vi "UE9 Frequency Output Stepping.vi"(8 "error in":errorcluster) -> (0 "error out":errorcluster)   [LabVIEW 2021]
panel:
  in  "Run Continuously":bool
  in  "Step Up and Down":bool
  out "Current Frequency":dbl=1.0 format="%.2f"
  in  "ms at each step":dbl=1000.0 format="%.2f"
  in  "stop":bool
  in  "Step Size":dbl=2000.0 format="%.2f"
  in  "Finish Frequency":dbl=10000.0 format="%.2f"
  in  "Start Frequency":dbl=2000.0 format="%.2f"
  in  "FirstFound":bool=TRUE
  in  "Address":string="1"
  in  "ConnectionType":u16(ring) items=["LJ_ctUSB", "LJ_ctETHERNET"]
  out "Error Message":string
  # "Demonstrates 1 channel of frequency output sweeping on FIO0."
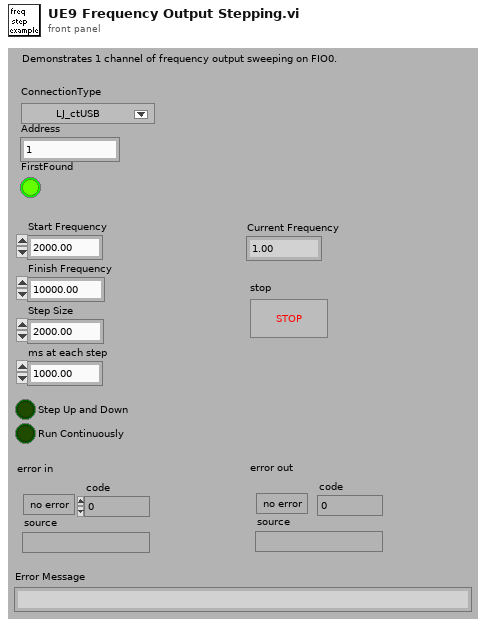
[diagram p1: front panel]
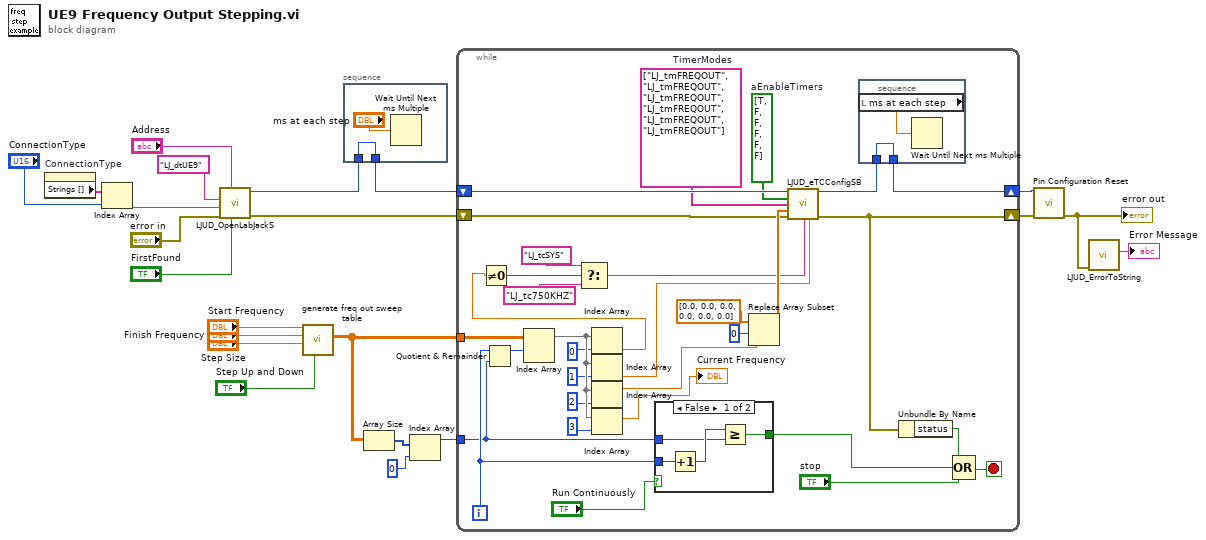
[diagram p0: block diagram]
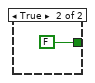
[diagram p2: hidden frame]
diagram:
  n1 = property on="ConnectionType" class="Ring (strict)"() -> ("Strings []"=w8:string[])  [unwired: 2 in, 2 out]
  n2 = Index Array(array=w8, index="ConnectionType") -> (element=w7:string)
  n3 = call "LJUD_OpenLabJackS.vi"("FirstFound"="FirstFound", "Address"="Address", "error in"="error in", "ConnectionType"=w7, "DeviceType"="LJ_dtUE9") -> ("error out"=w1:errorcluster, "Handle"=w2:i32)  [unwired: 4 in, 1 out]
  n4 = call "generate freq out sweep table.vi"("Step Up and Down"="Step Up and Down", "Step Size"="Step Size", "Finish Frequency"="Finish Frequency", "Start Frequency"="Start Frequency") -> ("Clock, ClockDivisor, FreqDivisor, Frequency"=w15:dbl[][])  [unwired: 7 in]
  n5 = stacked-sequence {
    tunnel: [w24] -> w10
    tunnel: w2 -> [w24]
    frame #0 {
      n6 = Wait Until Next ms Multiple(millisecond multiple="ms at each step") -> ()  [unwired: 1 out]
    }
  }
  n7 = Array Size(array=w15) -> (size(s)=w14:i32[])
  n8 = Index Array(array=w14, index=0 ("Index")) -> (element=w13:i32)
  n9 = while {
    tunnel: w13 -> [w46]
    shift-left: w1 -> [w38]
    shift-right: [w42] -> w4
    shift-left: w10 -> [w37]
    shift-right: [w50] -> w5
    tunnel: w15 -> [w49]
    i -> [w47]
    stop <- w54 stop-if-true
    w36 = bool[] [TRUE, FALSE, FALSE, FALSE, FALSE, FALSE]  # aEnableTimers
    w35 = string[] ["LJ_tmFREQOUT", "LJ_tmFREQOUT", "LJ_tmFREQOUT", "LJ_tmFREQOUT", "LJ_tmFREQOUT", "LJ_tmFREQOUT"]  # TimerModes
    n10 = Quotient & Remainder(x=w47, y=w46) -> (x-y*floor(x/y)=w45:i32)  [unwired: 1 out]
    n11 = Index Array(array=w49, index (row)=w45) -> (element=w33:dbl[])  [unwired: 1 in]
    n12 = Index Array(array=w33, index=0 ("Index")) -> (element=w28:dbl)
    n13 = Not Equal To 0?(x=w28) -> (x != 0?=w41:bool)
    n14 = Select(t="LJ_tcSYS", s=w41, f="LJ_tc750KHZ") -> (s? t:f=w34:string)
    n15 = Index Array(array=w33, index=1 ("Index")) -> (element=w27:dbl)
    n16 = Index Array(array=w33, index=2 ("Index")) -> (element=w26:dbl)
    n17 = Index Array(array=w33, index=3 ("Index")) -> (element=→"Current Frequency":dbl)
    n18 = case shown="False" "Run Continuously" {
      tunnel: [w60 FALSE] -> w51
      tunnel: w47 -> [w59 _]
      tunnel: w46 -> [w57 _]
      frame False {
        n19 = Increment(x=w59) -> (x+1=w58:i32)
        n20 = Greater Or Equal?(x=w58, y=w57) -> (x >= y?=w60:bool)
      }
      frame True {
      }
    }
    n21 = Replace Array Subset(array=dbl[] [0.0, 0.0, 0.0, 0.0, 0.0, 0.0] ("TimerValues"), new element=w26, index=0 ("Index")) -> (w44:dbl[])
    n22 = call "LJUD_eTCConfigSB.vi"("Handle In"=w37, "aEnableTimers"=w36, "aTimerModes"=w35, "aTimerValues"=w44, "error in"=w38, "TimerClockBase"=w34, "TimerClockDivisor"=w27) -> ("Handle Out"=w43:i32, "error out"=w42:errorcluster)  [unwired: 7 in]
    n23 = stacked-sequence {
      tunnel: [w63] -> w50
      tunnel: w43 -> [w63]
      frame #0 {
        n24 = local read "ms at each step"() -> (w62:dbl)
        n25 = Wait Until Next ms Multiple(millisecond multiple=w62) -> ()  [unwired: 1 out]
      }
    }
    n26 = Unbundle By Name(w42) -> ("status"=w53:bool)
    n27 = Compound Arithmetic op=OR(w53, w51, "stop") -> (w54:bool)
  }
  n28 = call "Pin Configuration Reset.vi"("error in"=w4, "Handle In"=w5) -> ("error out"=w3:errorcluster)  [unwired: 8 in, 1 out]
  "error out" <- w3
  n29 = call "LJUD_ErrorToString.vi"("error in"=w3) -> ("String"=→"Error Message":string)  [unwired: 10 in]
